vi "TargetToJSON.vi"(8 "error in":errorcluster, 9 "JSON Path":path, 10 "head in":refnum<data-value>, 11 "Target Obj":refnum<vi>) -> (0 "error out":errorcluster, 2 "Paths":cluster{"Path":path, "JSON Path":path}[](array[cluster]))   [LabVIEW 2017]
uses:
  Helpers/DirectoryMetadata/DirectoryMetadata.lvclass
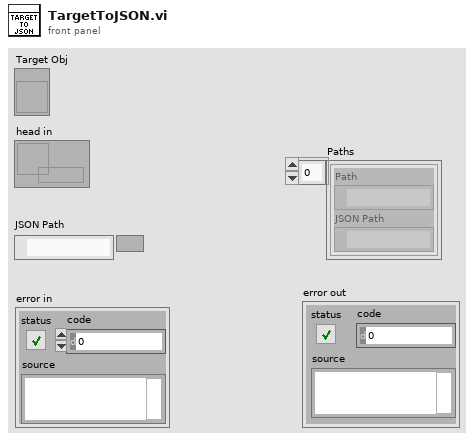
[diagram p1: front panel]
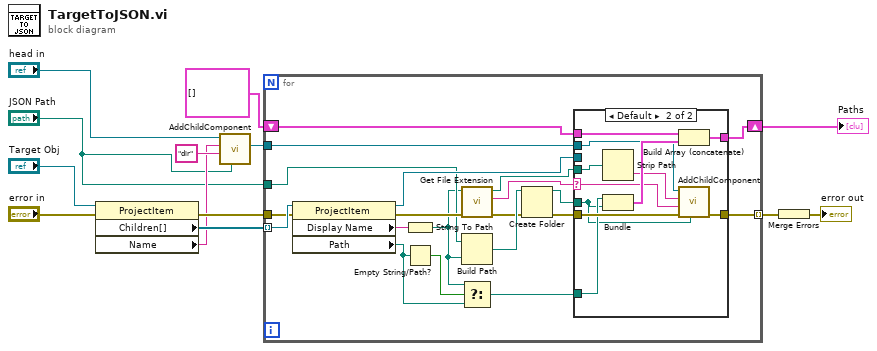
[diagram p0: block diagram]
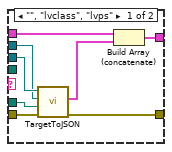
[diagram p2: hidden frame]
diagram:
  n1 = property class="ProjectItem"(reference="Target Obj", error in="error in") -> (error out=w10:errorcluster, "Children[]"=w11:refnum<vi>[], "Name"=w3:string)  [unwired: 1 out]
  n2 = call "AddChildComponent.vi"("Path"="JSON Path", "Type"="dir", "ID"=w3, "head in"="head in") -> ("child ref"=w2:refnum<data-value>)  [unwired: 5 in, 2 out]
  n3 = for {
    tunnel: w11 -> [w33] mode=indexing
    tunnel: w10 -> [w32]
    tunnel: [w31] -> w9 mode=indexing
    shift-right: [w27] -> w6
    shift-left: cluster{"Path":path, "JSON Path":path}[] [] ("Array") -> [w28]
    tunnel: w2 -> [w20]
    tunnel: "JSON Path" -> [w19]
    n4 = property class="ProjectItem"(reference=w33, error in=w32) -> (reference out=w26:refnum<vi>, error out=w30:errorcluster, "Display Name"=w23:string, "Path"=w22:path)
    n5 = String To Path(string=w23) -> (path=w18:path)
    n6 = Empty String/Path?(string/path=w22) -> (empty?=w24:bool)
    n7 = call <vilib>:"Get File Extension.vi"("error in (no error)"=w30, "file"=w18) -> ("error out"=w15:errorcluster, "lowercase file extension"=w29:string, "dup file"=w25:path)  [unwired: 5 in, 2 out]
    n8 = Build Path(base path=w19, name or relative path=w18) -> (appended path=w17:path)
    n9 = Select(t=w18, s=w24, f=w22) -> (s? t:f=w21:path)
    n10 = Create Folder(path (use dialog)=w17, error in=w15) -> (created path=w16:path, error out=w14:errorcluster)  [unwired: 1 in, 1 out]
    n11 = case shown="Default" w29 {
      selector: w29 -> [_ w49]
      tunnel: [w41 w45] -> w31
      tunnel: w14 -> [w40 w46]
      tunnel: w28 -> [w38 w52]
      tunnel: [w36 w51] -> w27
      tunnel: w21 -> [_ w43]
      tunnel: w26 -> [w39 _]
      tunnel: w20 -> [w35 w48]
      tunnel: w25 -> [_ w44]
      tunnel: w16 -> [w34 w42]
      frame "", "lvclass", "lvps" {
        n12 = call "TargetToJSON.vi"("error in"=w40, "JSON Path"=w34, "head in"=w35, "Target Obj"=w39) -> ("error out"=w41:errorcluster, "Paths"=w37:cluster{"Path":path, "JSON Path":path}[])  [unwired: 6 in]
        n13 = Build Array (concatenate)(w38, w37) -> (w36:cluster{"Path":path, "JSON Path":path}[])
      }
      frame Default {
        n14 = Strip Path(path=w44) -> (name=w47:string)  [unwired: 1 out]
        n15 = Bundle("Path"=w43, "created path"=w42) -> (w50:cluster{"Path":path, "created path":path})  [unwired: 1 in]
        n16 = Build Array (concatenate)(w52, w50) -> (w51:cluster{"Path":path, "created path":path}[])
        n17 = call "AddChildComponent.vi"("Path"=w42, "error in (no error)"=w46, "Type"=w49, "ID"=w47, "head in"=w48) -> ("error out"=w45:errorcluster)  [unwired: 4 in, 2 out]
      }
    }
  }
  "Paths" <- w6
  n18 = Merge Errors(w9) -> (→"error out":errorcluster)
